vi "Example.vi"() -> ()   [LabVIEW 2016]
panel:
  out "error out":errorcluster
  in  "LatitudeRef":string="South"
  in  "LongitudeRef":string="East"
  in  "AltitudeRef":string="Above Sea Level"
  in  "Altitude":string="100.700"
  in  "Longitude":string="90.0.0"
  in  "Latitude":string="10;37;11"
  out "Elapsed Time (s)":dbl
  out "Raw GPS Info":string
  out "standard error":string
  # "WRITE"
  # "READ"
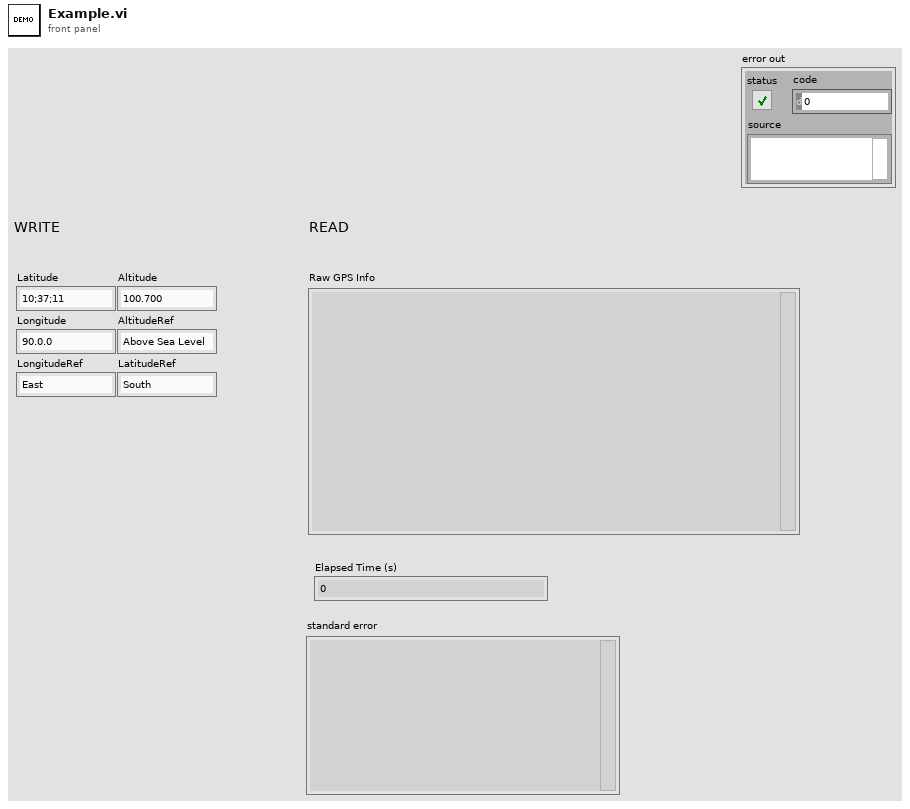
[diagram p1: front panel]
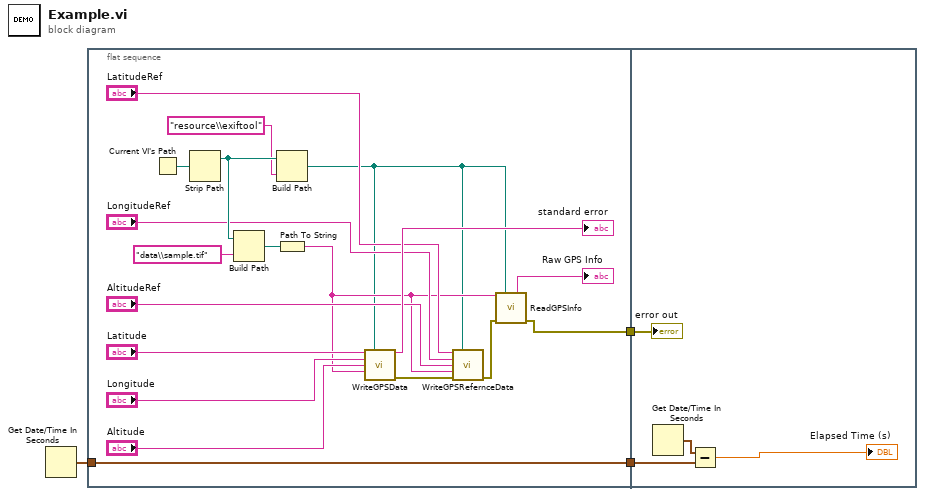
[diagram p0: block diagram]
diagram:
  n1 = Get Date/Time In Seconds() -> (seconds since 1Jan1904=w3:timestamp)
  n2 = flat-sequence {
    tunnel: w3 -> [w5]
    tunnel: [w5] -> w2
    tunnel: [w4] -> w1
    tunnel: w2 -> [w25]
    tunnel: w1 -> [w23]
    frame #0 {
      n3 = Current VI's Path() -> (path=w19:path)
      n4 = Strip Path(path=w19) -> (stripped path=w15:path)  [unwired: 1 out]
      n5 = Build Path(base path=w15, name or relative path="data\\sample.tif") -> (appended path=w17:path)
      n6 = Build Path(base path=w15, name or relative path="resource\\exiftool") -> (appended path=w7:path)
      n7 = Path To String(path=w17) -> (string=w9:string)
      n8 = call "WriteGPSData.vi"("Latitude"="Latitude", "ExifTool Path"=w7, "Longitude"="Longitude", "Altitude"="Altitude", "filepath"=w9) -> ("standard error"=→"standard error":string, "error out"=w10:errorcluster)  [unwired: 9 in]
      n9 = call "WriteGPSRefernceData.vi"("LatitudeRef"="LatitudeRef", "ExifTool Path"=w7, "LongitudeRef"="LongitudeRef", "AltitudeRef"="AltitudeRef", "filepath"=w9, "error in (no error)"=w10) -> ("error out"=w8:errorcluster)  [unwired: 8 in, 1 out]
      n10 = call "ReadGPSInfo.vi"("filepath"=w9, "ExifTool Path"=w7, "error in (no error)"=w8) -> ("Raw GPS Info"=→"Raw GPS Info":string, "error out"=w4:errorcluster)  [unwired: 5 in, 6 out]
    }
    frame #1 {
      n11 = Get Date/Time In Seconds() -> (seconds since 1Jan1904=w26:timestamp)
      n12 = Subtract(x=w26, y=w25) -> (x-y=→"Elapsed Time (s)":dbl)
      "error out" <- w23
    }
  }
